vi "HTTP.vi"() -> ()   [LabVIEW 2021]
uses:
  <vilib>/httpClient/POSTBuffer.vi
  <vilib>/httpClient/LabVIEWHTTPClient.lvlib
panel:
  out "length":i32
  out "error out 2":errorcluster
  out "headers":string
  out "error out":errorcluster
  out "data string 2":string
  out "data string":string
  in  "stop":bool
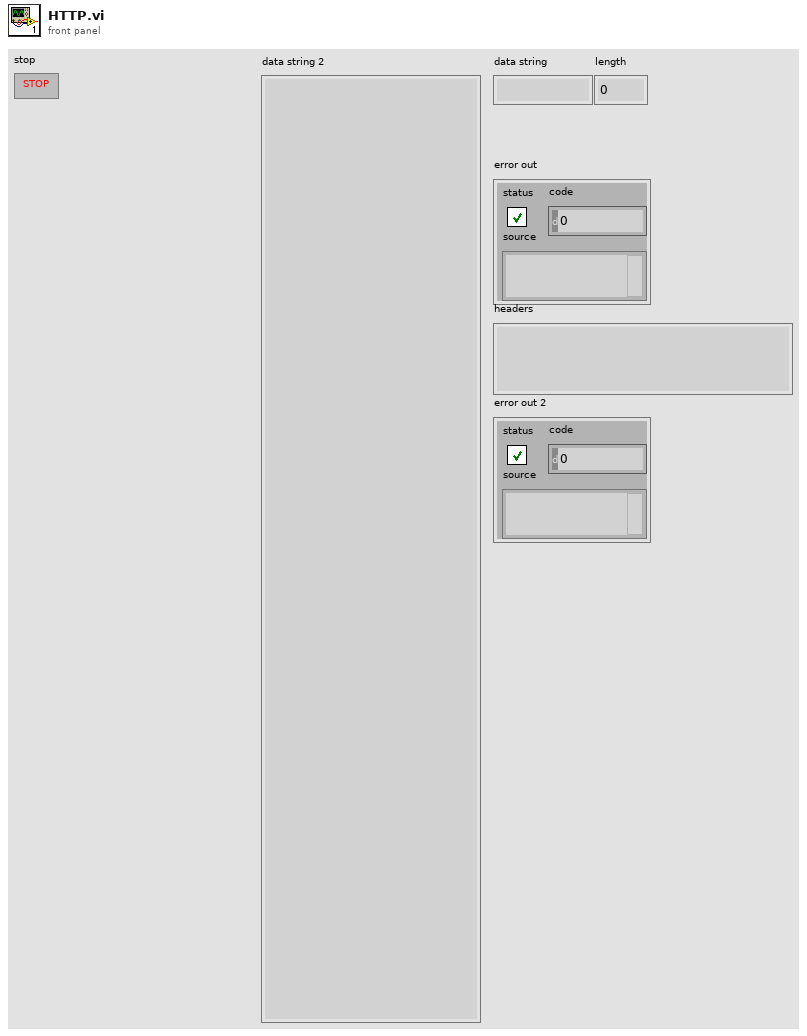
[diagram p1: front panel]
types:
  T1 = typedef "LabVIEWHTTPClient.lvlib/ClientHandle.ctl" = refnum<k1>
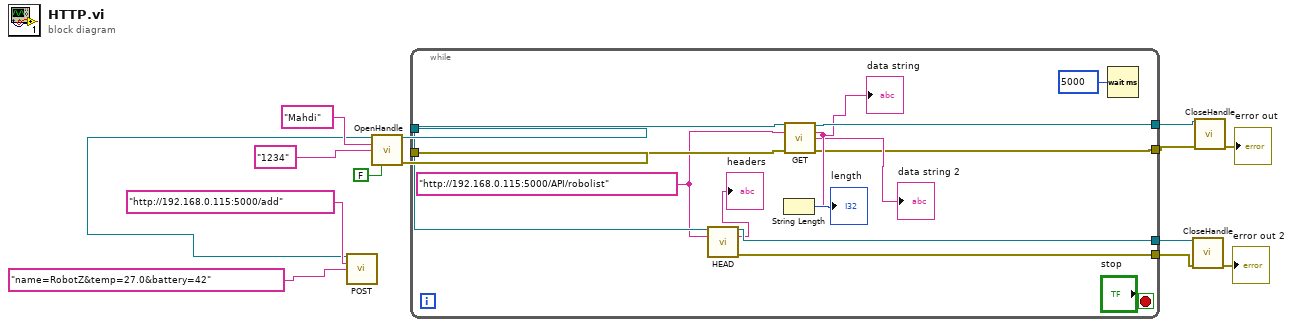
[diagram p0: block diagram]
diagram:
  n1 = call <vilib>:"OpenHandle.vi"("username"="Mahdi", "password"="1234", "verify server(true)"=FALSE) -> ("client handle out"=w1:T1, "error out"=w12:errorcluster)  [unwired: 11 in]
  n2 = call-poly <vilib>:"POST.vi"("client handle"=w1, "url"="http://192.168.0.115:5000/add", "buffer"="name=RobotZ&temp=27.0&battery=42") -> ()  [unwired: 9 in, 4 out]
  n3 = while {
    tunnel: w1 -> [w15]
    tunnel: w12 -> [w20]
    tunnel: [w16] -> w11
    tunnel: [w19] -> w10
    tunnel: [w24] -> w8
    tunnel: [w23] -> w7
    stop <- "stop" stop-if-true
    w14 = "http://192.168.0.115:5000/API/robolist" ("url")
    n4 = call <vilib>:"HEAD.vi"("client handle"=w15, "url"=w14) -> ("client handle out"=w23:T1, "headers"=→"headers":string, "error out"=w24:errorcluster)  [unwired: 11 in]
    n5 = call <vilib>:"GET.vi"("client handle"=w15, "url"=w14, "error in (no error)"=w20) -> ("client handle out"=w19:T1, "headers"=w18:string, "body"=→"data string 2":string, "error out"=w16:errorcluster)  [unwired: 9 in]
    "data string" <- w18
    n6 = String Length(string=w18) -> (length=→"length":i32)
    n7 = Wait (ms)(milliseconds to wait=u32 5000) -> ()  [unwired: 1 out]
  }
  n8 = call <vilib>:"CloseHandle.vi"("client handle"=w7, "error in (no error)"=w8) -> ("error out"=→"error out 2":errorcluster)  [unwired: 13 in]
  n9 = call <vilib>:"CloseHandle.vi"("client handle"=w10, "error in (no error)"=w11) -> ("error out"=→"error out":errorcluster)  [unwired: 13 in]
